vi "insert_column_into_array.vi"() -> ()   [LabVIEW 2021]
uses:
  <vilib>/Analysis/Matrix/Datatypes/RealMatrix.ctl
  <vilib>/Analysis/Matrix/NI_Matrix.lvlib
panel:
  in  "blank":dbl[](array[numeric])
  out "output":dbl[][](array[numeric])
  in  "loops":dbl
  in  "col index":dbl
  in  "mat":T1
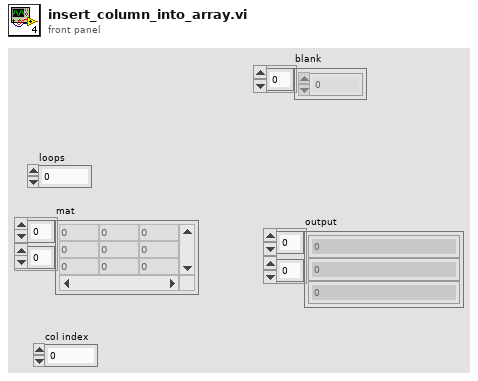
[diagram p1: front panel]
types:
  T1 = typedef "NI_Matrix.lvlib/RealMatrix.ctl" = dbl[][]
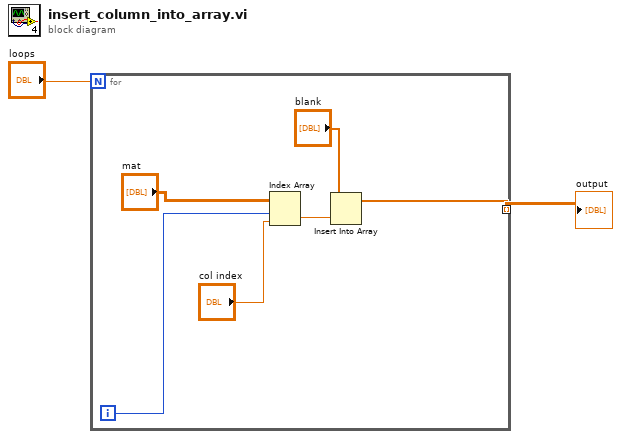
[diagram p0: block diagram]
diagram:
  n1 = for {
    N: "loops" -> [_]
    tunnel: [w3] -> w1 mode=indexing
    i -> [w4]
    n2 = Index Array(array="mat", index (row)=w4, index (col)="col index") -> (element=w7:dbl)
    n3 = Insert Into Array(array="blank", new element=w7) -> (w3:dbl[])  [unwired: 1 in]
  }
  "output" <- w1
